vi "bigcryo_T-control.vi"(5 "Ramp Mode":bool, 7 "Rate  [K/min]":dbl=2.0, 9 "VISA resource name out":refnum<visa-resource-name>="COM7", 11 "Set Sample Temp [K]":dbl=35.0) -> ()   [LabVIEW 2019]
panel:
  in  "VTI":dbl
  in  "Set VTI Explicit":bool
  out "PID":string
  out "String":string="+023.261E+0;+022.689E+0\n"
  in  "Auto PID":bool=TRUE
  out "D2":string="0"
  out "I2":string="10.095924"
  out "P2":string="150"
  out "D1":string="0"
  out "I1":string="40"
  out "P1":string="120"
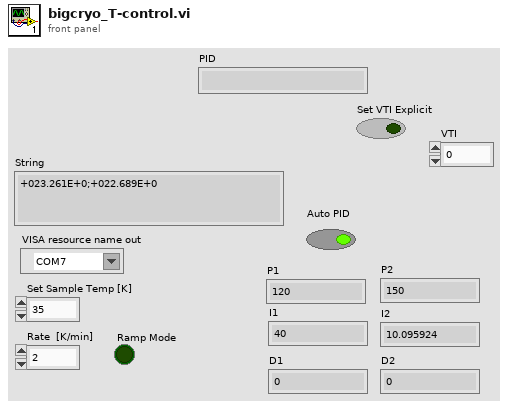
[diagram p1: front panel]
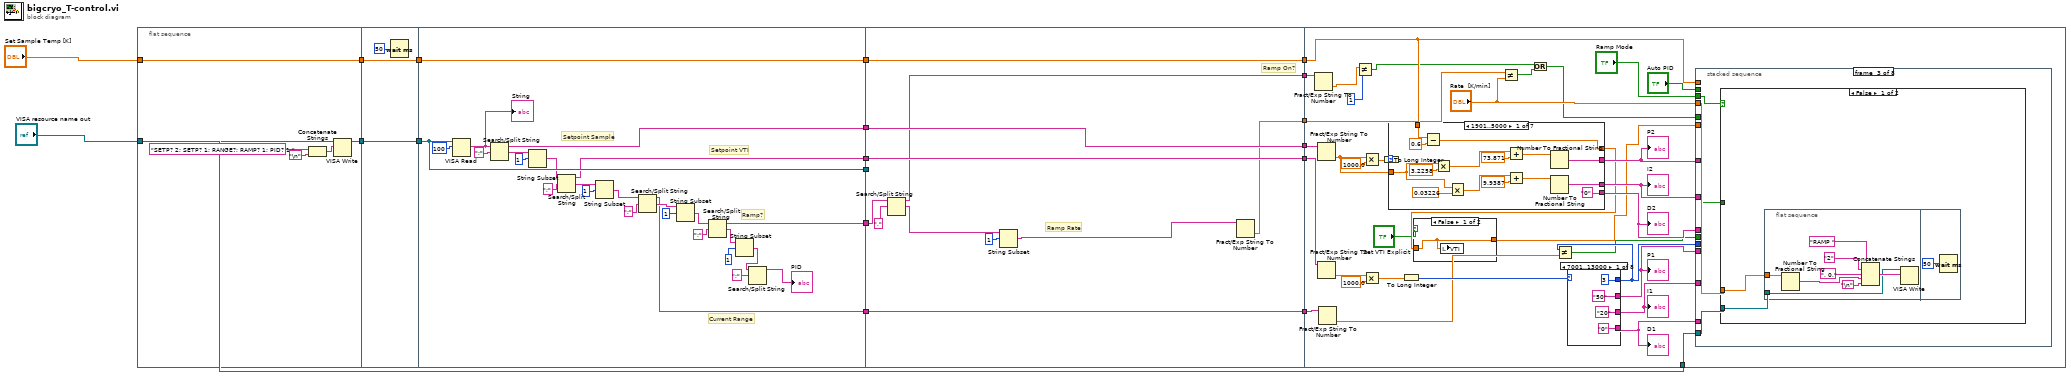
[diagram p0: block diagram]
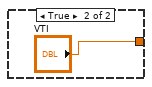
[diagram p2: hidden frame]
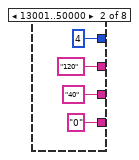
[diagram p3: hidden frame]
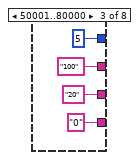
[diagram p4: hidden frame]
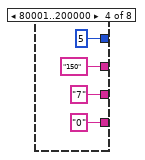
[diagram p5: hidden frame]
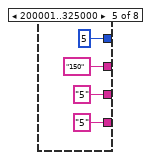
[diagram p6: hidden frame]
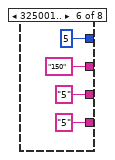
[diagram p7: hidden frame]
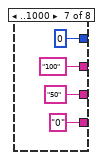
[diagram p8: hidden frame]
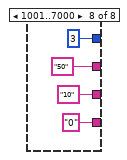
[diagram p9: hidden frame]
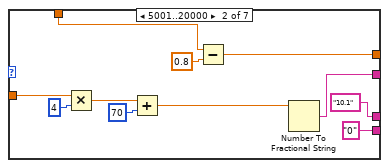
[diagram p10: hidden frame]
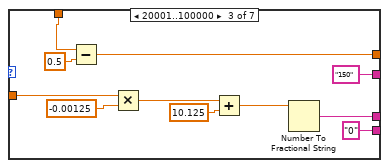
[diagram p11: hidden frame]
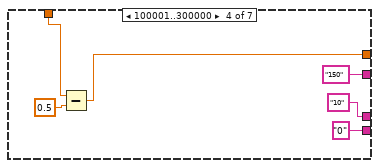
[diagram p12: hidden frame]
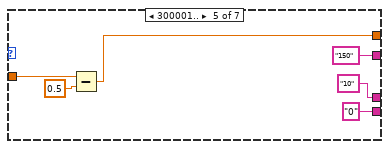
[diagram p13: hidden frame]
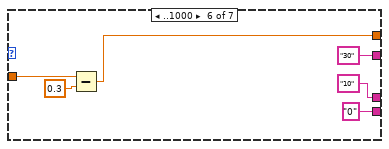
[diagram p14: hidden frame]
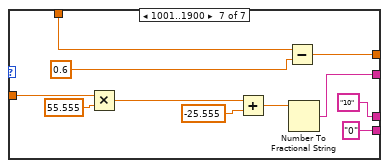
[diagram p15: hidden frame]
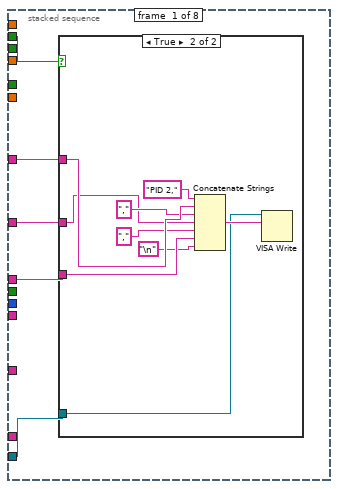
[diagram p16: hidden frame]
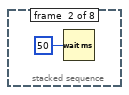
[diagram p18: hidden frame]
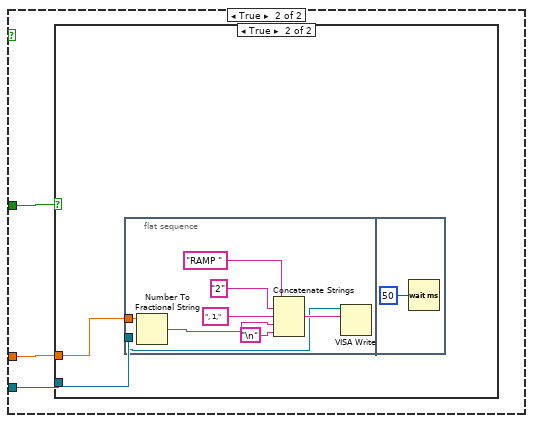
[diagram p19: hidden frame]
diagram:
  n1 = flat-sequence {
    tunnel: "VISA resource name out" -> [w20]
    tunnel: "Set Sample Temp [K]" -> [w24]
    tunnel: [w24] -> w11
    tunnel: [w19] -> w10
    tunnel: [w27] -> w13
    tunnel: [w26] -> w12
    tunnel: w11 -> [w27]
    tunnel: w10 -> [w26]
    tunnel: [w53] -> w15
    tunnel: [w51] -> w14
    tunnel: w13 -> [w53]
    tunnel: w12 -> [w51]
    tunnel: [w47] -> w9
    tunnel: [w41] -> w8
    tunnel: [w35] -> w4
    tunnel: [w33] -> w3
    tunnel: [w64] -> w16
    tunnel: [w63] -> w7
    tunnel: [w62] -> w6
    tunnel: [w61] -> w5
    tunnel: w15 -> [w64]
    tunnel: w14 -> [_]
    tunnel: w9 -> [w62]
    tunnel: w8 -> [w63]
    tunnel: w4 -> [w61]
    tunnel: w3 -> [w60]
    tunnel: [w58] -> w2
    tunnel: [w54] -> w1
    tunnel: "VISA resource name out" -> [w85]
    tunnel: w16 -> [w80]
    tunnel: w7 -> [w84]
    tunnel: w6 -> [w82]
    tunnel: w5 -> [w79]
    tunnel: w2 -> [w75]
    tunnel: w1 -> [w71]
    frame #0 {
      n2 = Concatenate Strings("SETP? 2; SETP? 1; RANGE?; RAMP? 1; PID? 1;" ("write buffer"), "\n") -> (w21:string)
      n3 = VISA Write(VISA resource name=w20, write buffer=w21) -> (VISA resource name out=w19:refnum<visa-resource-name>)  [unwired: 1 in, 2 out]
    }
    frame #1 {
      n4 = Wait (ms)(milliseconds to wait=50) -> ()  [unwired: 1 out]
    }
    frame #2 {
      # "Ramp?"
      # "Current Range"
      # "Setpoint VTI"
      # "Setpoint Sample"
      n5 = VISA Read(VISA resource name=w51, byte count=u32 100) -> (read buffer=w46:string)  [unwired: 1 in, 3 out]
      "String" <- w46
      n6 = Search/Split String(string=w46, search string/char (-)=";") -> (substring before match=w47:string, match + rest of string=w49:string)  [unwired: 1 in, 1 out]
      n7 = String Subset(string=w49, offset (0)=u32 1 ("byte count")) -> (substring=w42:string)  [unwired: 1 in]
      n8 = Search/Split String(string=w42, search string/char (-)=";") -> (substring before match=w41:string, match + rest of string=w45:string)  [unwired: 1 in, 1 out]
      n9 = String Subset(string=w45, offset (0)=u32 1 ("byte count")) -> (substring=w36:string)  [unwired: 1 in]
      n10 = Search/Split String(string=w36, search string/char (-)=";") -> (substring before match=w35:string, match + rest of string=w40:string)  [unwired: 1 in, 1 out]
      n11 = String Subset(string=w40, offset (0)=u32 1 ("byte count")) -> (substring=w34:string)  [unwired: 1 in]
      n12 = Search/Split String(string=w34, search string/char (-)=";") -> (substring before match=w33:string, match + rest of string=w32:string)  [unwired: 1 in, 1 out]
      n13 = String Subset(string=w32, offset (0)=u32 1 ("byte count")) -> (substring=w30:string)  [unwired: 1 in]
      n14 = Search/Split String(string=w30, search string/char (-)=";") -> (substring before match=→"PID":string)  [unwired: 1 in, 2 out]
    }
    frame #3 {
      # "Ramp Rate"
      # "Ramp On?"
      n15 = Search/Split String(string=w60, search string/char (-)=",") -> (substring before match=w58:string, match + rest of string=w56:string)  [unwired: 1 in, 1 out]
      n16 = String Subset(string=w56, offset (0)=u32 1 ("byte count")) -> (substring=w55:string)  [unwired: 1 in]
      n17 = Fract/Exp String To Number(string=w55) -> (number=w54:dbl)  [unwired: 3 in, 1 out]
    }
    frame #4 {
      n18 = Fract/Exp String To Number(string=w75) -> (number=w74:dbl)  [unwired: 3 in, 1 out]
      n19 = Fract/Exp String To Number(string=w82) -> (number=w81:dbl)  [unwired: 3 in, 1 out]
      n20 = Fract/Exp String To Number(string=w84) -> (number=w83:dbl)  [unwired: 3 in, 1 out]
      n21 = Fract/Exp String To Number(string=w79) -> (number=w78:dbl)  [unwired: 3 in, 1 out]
      n22 = Not Equal?(x=w74, y=1) -> (x != y?=w69:bool)
      n23 = Multiply(x=w81, y=1000.0) -> (x*y=w97:dbl)
      n24 = Multiply(x=w83, y=1000.0) -> (x*y=w94:dbl)
      n25 = To Long Integer(number=w97) -> (32bit integer=w98:i32)
      n26 = case shown="1901..5000" w98 {
        tunnel: w81 -> [w136 w155 w165 _ w181 w187 w190]
        tunnel: [w142 w154 w164 w175 w180 w186 w196] -> w67
        tunnel: [w144 w153 "150" "150" "150" "30" w194] -> w89
        tunnel: [w135 "10.1" w162 "10" "10" "10" "10"] -> w88
        tunnel: ["0" "0" "0" "0" "0" "0" "0"] -> w87
        tunnel: w80 -> [w134 w149 w160 w171 _ _ w189]
        frame 1901..5000 {
          n27 = Subtract(x=w134, y=0.6) -> (x-y=w142:dbl)
          n28 = Multiply(x=w136, y=3.2258) -> (x*y=w146:dbl)
          n29 = Multiply(x=w136, y=0.03226) -> (x*y=w138:dbl)
          n30 = Add(x=w146, y=73.871) -> (x+y=w145:dbl)
          n31 = Add(x=w138, y=9.9387) -> (x+y=w137:dbl)
          n32 = Number To Fractional String(number=w145) -> (F-format string=w144:string)  [unwired: 3 in]
          n33 = Number To Fractional String(number=w137) -> (F-format string=w135:string)  [unwired: 3 in]
        }
        frame 5001..20000 {
          n34 = Multiply(x=w155, y=4) -> (x*y=w157:dbl)
          n35 = Add(x=w157, y=70) -> (x+y=w156:dbl)
          n36 = Subtract(x=w149, y=0.8) -> (x-y=w154:dbl)
          n37 = Number To Fractional String(number=w156) -> (F-format string=w153:string)  [unwired: 3 in]
        }
        frame 20001..100000 {
          n38 = Subtract(x=w160, y=0.5) -> (x-y=w164:dbl)
          n39 = Multiply(x=w165, y=-0.00125) -> (x*y=w168:dbl)
          n40 = Add(x=w168, y=10.125) -> (x+y=w167:dbl)
          n41 = Number To Fractional String(number=w167) -> (F-format string=w162:string)  [unwired: 3 in]
        }
        frame 100001..300000 {
          n42 = Subtract(x=w171, y=0.5) -> (x-y=w175:dbl)
        }
        frame 300001.. {
          n43 = Subtract(x=w181, y=0.5) -> (x-y=w180:dbl)
        }
        frame ..1000 {
          n44 = Subtract(x=w187, y=0.3) -> (x-y=w186:dbl)
        }
        frame 1001..1900 {
          n45 = Multiply(x=w190, y=55.555) -> (x*y=w197:dbl)
          n46 = Add(x=w197, y=-25.555) -> (x+y=w195:dbl)
          n47 = Subtract(x=w189, y=0.6) -> (x-y=w196:dbl)
          n48 = Number To Fractional String(number=w195) -> (F-format string=w194:string)  [unwired: 3 in]
        }
      }
      "P2" <- w89
      "I2" <- w88
      "D2" <- w87
      n49 = To Long Integer(number=w94) -> (32bit integer=w93:i32)
      n50 = case shown="False" "Set VTI Explicit" {
        tunnel: w67 -> [w100 _]
        tunnel: [w100 "VTI"] -> w65
        frame False {
          n51 = local write "VTI"(w100) -> ()
        }
        frame True {
        }
      }
      n52 = Not Equal?(x=w71, y="Rate  [K/min]") -> (x != y?=w70:bool)
      n53 = Or(x=w69, y=w70) -> (x .or. y?=w68:bool)
      n54 = case shown="7001..13000" w93 {
        tunnel: [3 4 5 5 5 5 0 3] -> w77
        tunnel: ["50" "120" "100" "150" "150" "150" "100" "50"] -> w92
        tunnel: ["20" "40" "20" "7" "5" "5" "50" "10"] -> w91
        tunnel: ["0" "0" "0" "0" "5" "5" "0" "0"] -> w90
        frame 7001..13000 {
        }
        frame 13001..50000 {
        }
        frame 50001..80000 {
        }
        frame 80001..200000 {
        }
        frame 200001..325000 {
        }
        frame 325001.. {
        }
        frame ..1000 {
        }
        frame 1001..7000 {
        }
      }
      "P1" <- w92
      "I1" <- w91
      "D1" <- w90
      n55 = Not Equal?(x=w77, y=w78) -> (x != y?=w76:bool)
      n56 = stacked-sequence {
        tunnel: w85 -> [w201 _ w218 w245 w259 w274 w287 w316]
        tunnel: w65 -> [_ _ _ _ _ _ _ w315]
        tunnel: "Rate  [K/min]" -> [_ _ w217 _ _ _ w289 _]
        tunnel: w89 -> [w204 _ _ _ _ _ _ _]
        tunnel: w88 -> [w203 _ _ _ _ _ _ _]
        tunnel: w87 -> [w202 _ _ _ _ _ _ _]
        tunnel: "Ramp Mode" -> [_ _ w216 _ _ _ w288 _]
        tunnel: w80 -> [_ _ _ w244 _ _ _ _]
        tunnel: w77 -> [_ _ _ _ _ w275 _ _]
        tunnel: w92 -> [_ _ _ _ w258 _ _ _]
        tunnel: w91 -> [_ _ _ _ w257 _ _ _]
        tunnel: w90 -> [_ _ _ _ w256 _ _ _]
        tunnel: "Auto PID" -> [w200 _ _ _ w255 _ _ _]
        tunnel: w76 -> [_ _ _ _ _ w276 _ _]
        tunnel: w68 -> [_ _ w215 _ _ _ w286 _]
        frame #0 {
          n57 = case shown="True" w200 {
            tunnel: w204 -> [_ w211]
            tunnel: w203 -> [_ w209]
            tunnel: w202 -> [_ w207]
            tunnel: w201 -> [_ w205]
            frame False {
            }
            frame True {
              n58 = Concatenate Strings("PID 2," ("write buffer"), w211, "," ("write buffer"), w209, "," ("write buffer"), w207, "\n") -> (w213:string)
              n59 = VISA Write(VISA resource name=w205, write buffer=w213) -> ()  [unwired: 1 in, 3 out]
            }
          }
        }
        frame #1 {
          n60 = Wait (ms)(milliseconds to wait=u32 50) -> ()  [unwired: 1 out]
        }
        frame #2 {
          n61 = case shown="False" w216 {
            tunnel: w218 -> [w220 w232]
            tunnel: w217 -> [w219 w231]
            tunnel: w215 -> [_ w230]
            frame False {
              n62 = flat-sequence {
                tunnel: w220 -> [w222]
                tunnel: w219 -> [w221]
                frame #0 {
                  n63 = Number To Fractional String(number=w221) -> (F-format string=w225:string)  [unwired: 3 in]
                  n64 = Concatenate Strings("RAMP " ("write buffer"), "2" ("write buffer"), ", 0," ("write buffer"), w225, "\n") -> (w228:string)
                  n65 = VISA Write(VISA resource name=w222, write buffer=w228) -> ()  [unwired: 1 in, 3 out]
                }
                frame #1 {
                  n66 = Wait (ms)(milliseconds to wait=u32 50) -> ()  [unwired: 1 out]
                }
              }
            }
            frame True {
              n67 = case shown="True" w230 {
                tunnel: w232 -> [_ w234]
                tunnel: w231 -> [_ w233]
                frame False {
                }
                frame True {
                  n68 = flat-sequence {
                    tunnel: w234 -> [w240]
                    tunnel: w233 -> [w239]
                    frame #0 {
                      n69 = Number To Fractional String(number=w239) -> (F-format string=w237:string)  [unwired: 3 in]
                      n70 = Concatenate Strings("RAMP " ("write buffer"), "2" ("write buffer"), ", 1," ("write buffer"), w237, "\n") -> (w242:string)
                      n71 = VISA Write(VISA resource name=w240, write buffer=w242) -> ()  [unwired: 1 in, 3 out]
                    }
                    frame #1 {
                      n72 = Wait (ms)(milliseconds to wait=u32 50) -> ()  [unwired: 1 out]
                    }
                  }
                }
              }
            }
          }
        }
        frame #3 {
          n73 = flat-sequence {
            tunnel: w245 -> [w252]
            tunnel: w244 -> [w246]
            frame #0 {
              n74 = Number To Fractional String(number=w246) -> (F-format string=w250:string)  [unwired: 3 in]
              n75 = Concatenate Strings("SETP " ("write buffer"), "2" ("write buffer"), "," ("write buffer"), w250, "\n") -> (w253:string)
              n76 = VISA Write(VISA resource name=w252, write buffer=w253) -> ()  [unwired: 1 in, 3 out]
            }
            frame #1 {
              n77 = Wait (ms)(milliseconds to wait=u32 50) -> ()  [unwired: 1 out]
            }
          }
        }
        frame #4 {
          n78 = case shown="True" w255 {
            tunnel: w259 -> [_ w263]
            tunnel: w258 -> [_ w262]
            tunnel: w257 -> [_ w261]
            tunnel: w256 -> [_ w260]
            frame False {
            }
            frame True {
              n79 = flat-sequence {
                tunnel: w263 -> [w267]
                tunnel: w262 -> [w266]
                tunnel: w261 -> [w265]
                tunnel: w260 -> [w264]
                frame #0 {
                  n80 = Concatenate Strings("PID 1," ("write buffer"), w266, "," ("write buffer"), w265, "," ("write buffer"), w264, "\n") -> (w271:string)
                  n81 = VISA Write(VISA resource name=w267, write buffer=w271) -> ()  [unwired: 1 in, 3 out]
                }
                frame #1 {
                  n82 = Wait (ms)(milliseconds to wait=u32 50) -> ()  [unwired: 1 out]
                }
              }
            }
          }
        }
        frame #5 {
          n83 = case shown="True" w276 {
            tunnel: w275 -> [_ w278]
            tunnel: w274 -> [_ w277]
            frame False {
            }
            frame True {
              n84 = flat-sequence {
                tunnel: w278 -> [w282]
                tunnel: w277 -> [w279]
                frame #0 {
                  n85 = Number To Fractional String(number=w282) -> (F-format string=w283:string)  [unwired: 3 in]
                  n86 = Concatenate Strings("RANGE " ("write buffer"), w283, "\n") -> (w284:string)
                  n87 = VISA Write(VISA resource name=w279, write buffer=w284) -> ()  [unwired: 1 in, 3 out]
                }
                frame #1 {
                  n88 = Wait (ms)(milliseconds to wait=u32 50) -> ()  [unwired: 1 out]
                }
              }
            }
          }
        }
        frame #6 {
          n89 = case shown="True" w288 {
            tunnel: w289 -> [w290 w303]
            tunnel: w287 -> [w291 w302]
            tunnel: w286 -> [_ w301]
            frame False {
              n90 = flat-sequence {
                tunnel: w291 -> [w293]
                tunnel: w290 -> [w292]
                frame #0 {
                  n91 = Number To Fractional String(number=w292) -> (F-format string=w296:string)  [unwired: 3 in]
                  n92 = Concatenate Strings("RAMP " ("write buffer"), "1" ("write buffer"), ", 0," ("write buffer"), w296, "\n") -> (w299:string)
                  n93 = VISA Write(VISA resource name=w293, write buffer=w299) -> ()  [unwired: 1 in, 3 out]
                }
                frame #1 {
                  n94 = Wait (ms)(milliseconds to wait=u32 50) -> ()  [unwired: 1 out]
                }
              }
            }
            frame True {
              n95 = case shown="False" w301 {
                tunnel: w303 -> [_ w305]
                tunnel: w302 -> [_ w304]
                frame False {
                }
                frame True {
                  n96 = flat-sequence {
                    tunnel: w305 -> [w307]
                    tunnel: w304 -> [w306]
                    frame #0 {
                      n97 = Number To Fractional String(number=w307) -> (F-format string=w310:string)  [unwired: 3 in]
                      n98 = Concatenate Strings("RAMP " ("write buffer"), "1" ("write buffer"), ", 1," ("write buffer"), w310, "\n") -> (w313:string)
                      n99 = VISA Write(VISA resource name=w306, write buffer=w313) -> ()  [unwired: 1 in, 3 out]
                    }
                    frame #1 {
                      n100 = Wait (ms)(milliseconds to wait=u32 50) -> ()  [unwired: 1 out]
                    }
                  }
                }
              }
            }
          }
        }
        frame #7 {
          n101 = flat-sequence {
            tunnel: w316 -> [w318]
            tunnel: w315 -> [w317]
            frame #0 {
              n102 = Number To Fractional String(number=w317) -> (F-format string=w322:string)  [unwired: 3 in]
              n103 = Concatenate Strings("SETP " ("write buffer"), "1" ("write buffer"), "," ("write buffer"), w322, "\n") -> (w324:string)
              n104 = VISA Write(VISA resource name=w318, write buffer=w324) -> ()  [unwired: 1 in, 3 out]
            }
            frame #1 {
              n105 = Wait (ms)(milliseconds to wait=u32 50) -> ()  [unwired: 1 out]
            }
          }
        }
      }
    }
  }
